vi "CRYProject Editor PIC Send Event to Main.vi"(9 "nData":i32, 10 "sData":string="GVSMAIN_ACTION", 11 "sEventName":string="GVSMAIN_ACTION") -> ()   [LabVIEW 2013]
uses:
  CRYProject Editor Global.vi
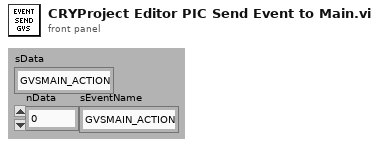
[diagram p1: front panel]
types:
  T1 = cluster{"EventName":string, "Arg1":string, "Numeric":u16, "Numeric 2":u16, "AddSteps ":refnum<vi>, "Arg1 2":string, "Arg1 3":string, "Boolean":bool}
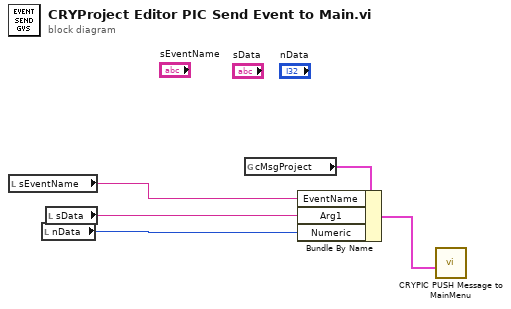
[diagram p0: block diagram]
diagram:
  n1 = local read "sEventName"() -> (w4:string)
  n2 = local read "nData"() -> (w3:i32)
  n3 = local read "sData"() -> (w5:string)
  n4 = global read "CRYProject Editor Global.vi" "cMsgProject"() -> (w2:T1)
  n5 = Bundle By Name(cluster=w2, "EventName"=w4, "Arg1"=w5, "Numeric"=w3) -> (w1:T1)
  n6 = call "CRYPIC PUSH Message to MainMenu.vi"("cMsgProject"=w1) -> ()  [unwired: 11 in]
